vi "Write JSON Config.vi"(6 "Pretty Print?":bool, 8 "error in (no error)":errorcluster, 11 "Const_Str in":refnum<class "Const_Str.lvclass">) -> (0 "error out":errorcluster, 2 "JSON":string, 3 "Const_Str out":refnum<class "Const_Str.lvclass">)   [LabVIEW 2021, in "Const_Str.lvclass"]
uses:
  Const_Str.lvclass
  C:/Program Files (x86)/National Instruments/LabVIEW 2021/vi.lib/TSA/Abstract Data Classes/Abs_Types/Type/Abs_Type.lvclass
  Const_Str.lvclass/Const_Str.ctl
  1408ddf9-9f8e-4de8-8927-e31d907d641d.vi
  <vilib>/Utility/LVClass/Get LV Class Name.vi
  <vilib>/JDP Science/JSONtext/Variant to JSON Text.vi
  <vilib>/JDP Science/JSONtext/Set Multiple Object Items.vi
  <vilib>/JDP Science/JSONtext/LVClass Serializer/JSONtext LVClass Serializer.lvclass
  Abs_Types/String/Abs_String.lvclass
  Abs_Types/Type/Abs_Type.lvclass
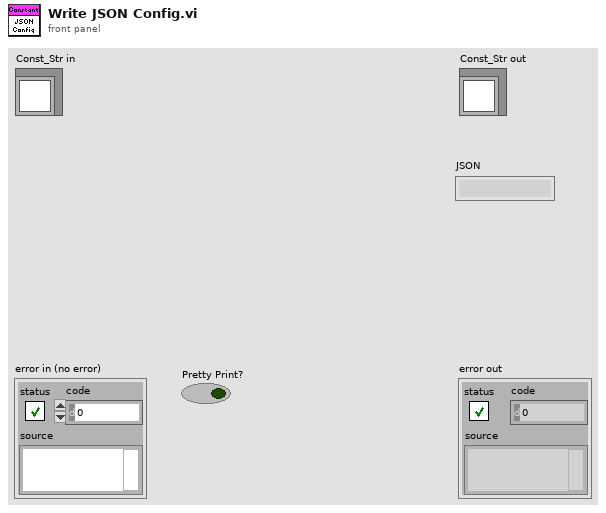
[diagram p1: front panel]
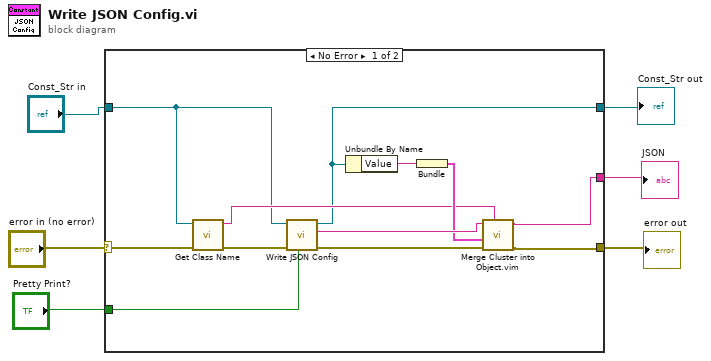
[diagram p0: block diagram]
diagram:
  n1 = case shown="No Error" "error in (no error)" {
    selector: "error in (no error)" -> [w17 w20]
    tunnel: [w11 w20] -> w4
    tunnel: [w12 _] -> w1
    tunnel: [w8 w19] -> w5
    tunnel: "Const_Str in" -> [w10 w19]
    tunnel: "Pretty Print?" -> [w7 _]
    frame No Error {
      n2 = call "Get Class Name.vi"("error in (no error)"=w17, "Abs_Type in"=w10) -> ("error out"=w18:errorcluster, "class name"=w13:string)  [unwired: 8 in]
      n3 = call-parent "Write JSON Config.vi"("Pretty Print?"=w7, "error in (no error)"=w18, "Abs_Type in"=w10) -> ("error out"=w16:errorcluster, "JSON"=w15:string, "Abs_Type out"=w8:refnum<class "Const_Str.lvclass">)  [unwired: 6 in]
      n4 = Unbundle By Name(w8) -> ("Value"=w9:string)
      n5 = Bundle("Value"=w9) -> (w14:cluster{"Value":string})  [unwired: 1 in]
      n6 = call "Merge Cluster into Object.vim"("$Path or Item Name"=w13, "error in (no error)"=w16, "Any Cluster"=w14, "JSON"=w15) -> ("error out"=w11:errorcluster, "<JSON>"=w12:string)  [unwired: 5 in]
    }
    frame Error {
    }
  }
  "error out" <- w4
  "Const_Str out" <- w5
  "JSON" <- w1
